vi "Main.vi"() -> ()   [LabVIEW 2017, in "Logger.lvlib"]
doc: "This template is based off of the Queued Message Handler design pattern and the Queued Message Handler project template that ships with LabVIEW.\n\nThe main difference is that the queue is private to this module and communication between modules is performed via Broadcast and Request events.\n\nRequest events are wrapped in public API methods and are handled in the Event Handling Loop (EHL) of this VI. Any module can register for Broadcast events sent by this module. The EHL generates messages based on user interface actions.\n\nThe Message Handling Loop (MHL) processes messages generated by the EHL, or by other messages. The messages are string values, so new messages can be added easily to the Message Cases case structure in the MHL. Each message cluster can also provide an optional value for Message Data, which is a variant that can be converted to whatever message-specific data is required.\n_____\nBased on Delacor QMH Project Template 4.0.0.47.\n_____\nBased on Delacor QMH Project Template 4.1.0.56."
uses:
  Logger.lvlib
  <vilib>/Delacor/Delacor QMH/Libraries/Module Admin_class/Delacor_lib_QMH_Module Admin.lvclass
  Module Data--cluster.ctl
  Stop Argument--cluster.ctl
  <vilib>/Delacor/Delacor QMH/Libraries/Module Admin_class/Delacor_lib_QMH_Module Admin.lvclass/Delacor_lib_QMH_Module Admin.ctl
  Initialize File Argument--cluster.ctl
  Initialize File (Reply Payload)--cluster.ctl
  Log Data Argument--cluster.ctl
  Stop Logging Argument--cluster.ctl
  Settings Editor/Update Application Settings (Reply Payload)--cluster.ctl
  Settings Editor/Settings--cluster.ctl
  CML Shared/Signal Type--enum.ctl
  CML Shared/Calibration Values--cluster.ctl
  <vilib>/Utility/miscctls.llb/LVPointTypeDef.ctl
  <vilib>/Delacor/Delacor QMH/Libraries/Module Admin_class/Delacor_lib_QMH_Get External Launch.vi
  <vilib>/Delacor/Delacor QMH/Libraries/Message Queue_class/Delacor_lib_QMH_Enqueue Message (Single).vi
  <vilib>/Utility/error.llb/Error Cluster From Error Code.vi
  <vilib>/ErrorRing/Error Ring.xnode
  <vilib>/Delacor/Delacor QMH/Libraries/Message Queue_class/Delacor_lib_QMH_Message Queue.lvclass
  Settings Editor/Settings Editor.lvlib
  CML Shared/CML Shared.lvlib
panel:
  out "Settings":T1
  out "error out":errorcluster
  in  "Module Admin":refnum<class "Delacor_lib_QMH_Module Admin.lvclass">
  # "This is a headless module. \nShow its panel to confirm that the Settings are updated correctly and other debugging tasks.\nUse the Settings Editor to change the settings for this module."
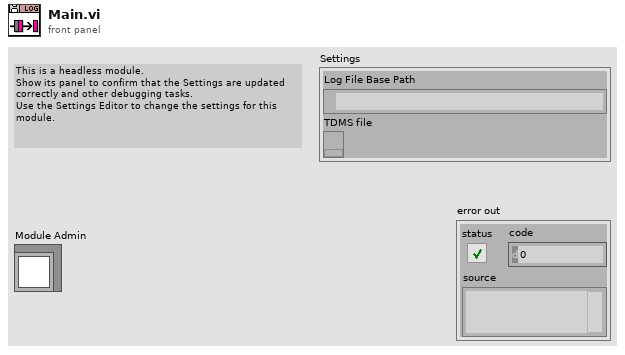
[diagram p1: front panel]
types:
  T1 = typedef "Logger.lvlib/Module Data--cluster.ctl" = cluster{"Log File Base Path":path, "TDMS file":refnum<k34>}
  T2 = typedef "Settings Editor.lvlib/Broadcast Events--cluster.ctl" = cluster{"Module Did Init":refnum<user-event>, "Status Updated":refnum<user-event>, "Error Reported":refnum<user-event>, "Module Did Stop":refnum<user-event>, "Update Module Execution Status":refnum<user-event>, "Application Settings Updated":refnum<user-event>}
  T3 = typedef "Logger.lvlib/Request Events--cluster.ctl" = cluster{"Stop Module":refnum<user-event>, "Show Panel":refnum<user-event>, "Hide Panel":refnum<user-event>, "Get Module Execution Status":refnum<user-event>, "Show Diagram":refnum<user-event>, "Stop Logging":refnum<user-event>, "Log Data":refnum<user-event>, "Initialize File":refnum<user-event>}
  T4 = enum32{"invalid lock state", "Not Locked", "Locked (No Password)", "Password-protected"}
  T5 = typedef "Logger.lvlib/Stop Argument--cluster.ctl" = cluster{"Origin":string, "Exit via Stop Module Req?":bool, "Wait for Module to stop?":bool}
  T6 = typedef "Logger.lvlib/Initialize File Argument--cluster.ctl" = cluster{"Wait Notifier":refnum<notifier>, "wait for reply":bool}
  T7 = typedef "Logger.lvlib/Log Data Argument--cluster.ctl" = cluster{"Waveforms":waveform(dbl)[]}
  T8 = typedef "Logger.lvlib/Stop Logging Argument--cluster.ctl" = cluster{"Boolean":bool}
  T9 = typedef "Settings Editor.lvlib/Update Application Settings (Reply Payload)--cluster.ctl" = cluster{"Settings":T10, "Update Settings_error":errorcluster}
  T10 = typedef "Settings Editor.lvlib/Settings--cluster.ctl" = cluster{"Signal Type":T11, "Calibration Array":T12[], "Log File Base Path":path}
  T11 = typedef "CML Shared.lvlib/Signal Type--enum.ctl" = enum16{"Sine Wave", "Square with Noise"}
  T12 = typedef "CML Shared.lvlib/Calibration Values--cluster.ctl" = cluster{"Slope":dbl, "Offset":dbl}
  T13 = typedef "LVPointTypeDef.ctl" = cluster{"Horizontal":i16, "Vertical":i16}
  T14 = enum32{"Invalid", "Standard", "Closed", "Hidden", "Minimized", "Maximized"}
  T15 = typedef "Logger.lvlib/Initialize File (Reply Payload)--cluster.ctl" = cluster{"File Path":path, "Initialize File_error":errorcluster}
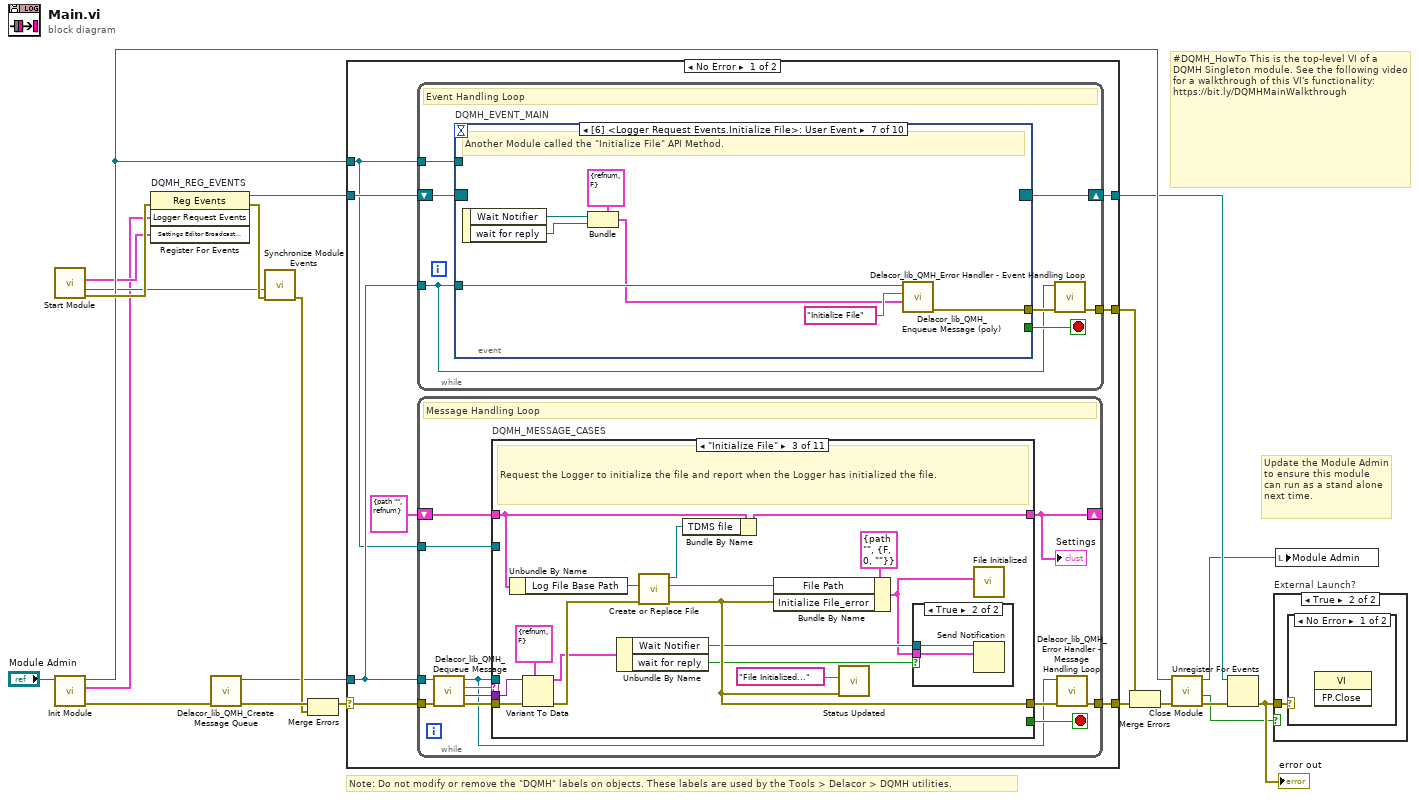
[diagram p0: block diagram]
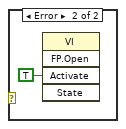
[diagram p3: hidden frame]
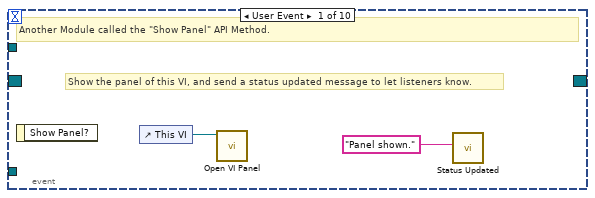
[diagram p4: hidden frame]
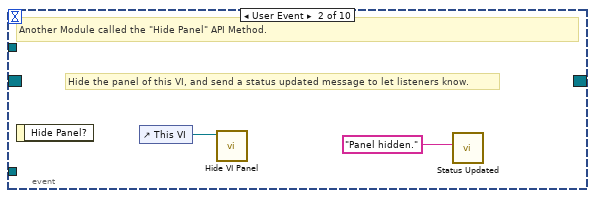
[diagram p5: hidden frame]
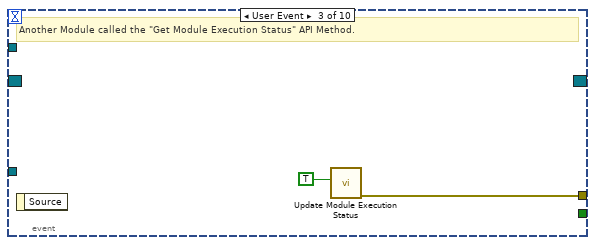
[diagram p6: hidden frame]
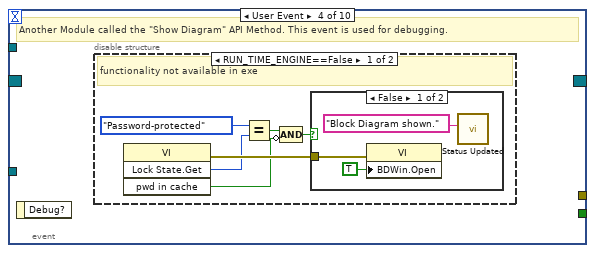
[diagram p7: hidden frame]
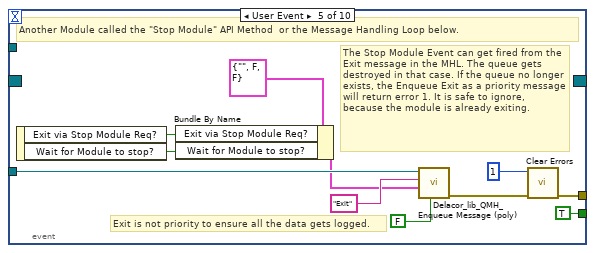
[diagram p10: hidden frame]
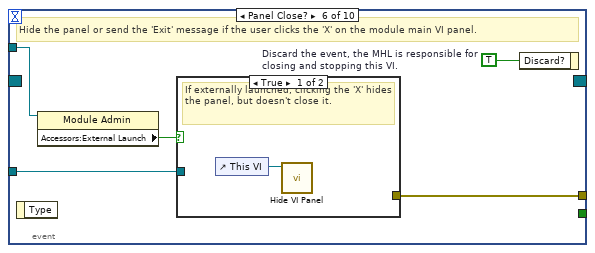
[diagram p11: hidden frame]
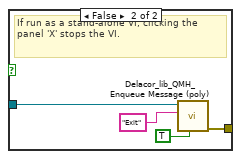
[diagram p12: hidden frame]
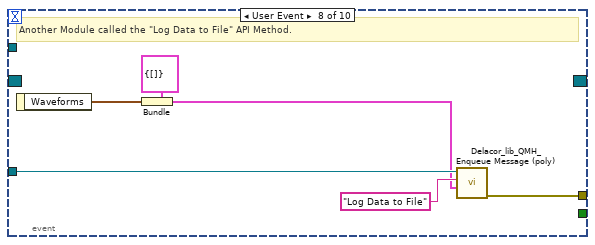
[diagram p13: hidden frame]
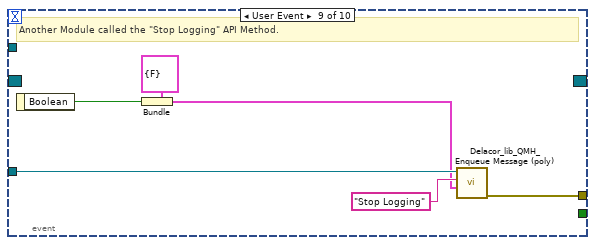
[diagram p14: hidden frame]
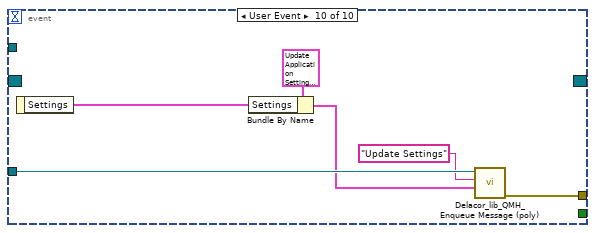
[diagram p15: hidden frame]
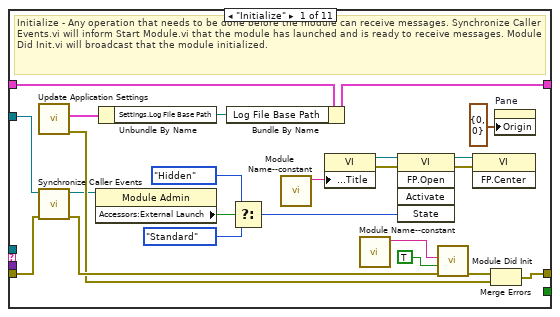
[diagram p16: hidden frame]
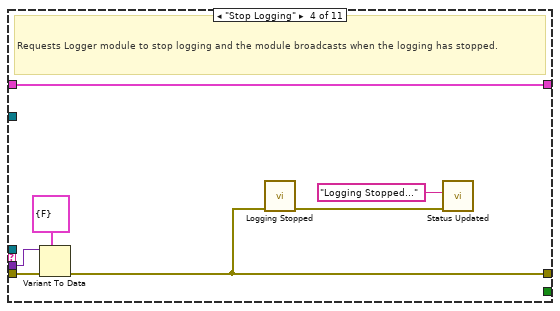
[diagram p19: hidden frame]
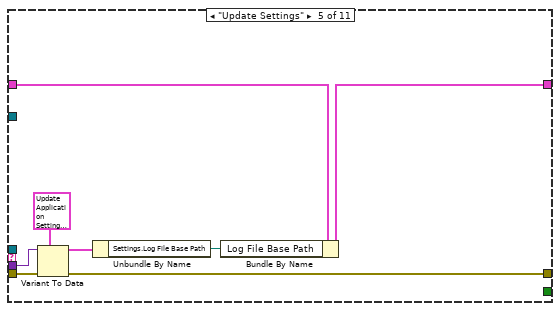
[diagram p20: hidden frame]
diagram:
  # "#DQMH_HowTo This is the top-level VI of a DQMH Singleton module. See the following video for a walkthrough of this VI's functionality: https://bit.ly/DQMHMainWalkthrough"
  # "Note: Do not modify or remove the \"DQMH\" labels on objects. These labels are used by the Tools > Delacor > DQMH utilities."
  # "Update the Module Admin to ensure this module can run as a stand alone next time."
  n1 = call "Start Module.vi"() -> ("error out"=w13:errorcluster, "Wait for Event Sync?"=w3:bool, "Settings Editor Broadcast Events"=w2:T2)  [unwired: 8 in, 1 out]
  n2 = call "Init Module.vi"("Singleton Module Admin in"="Module Admin") -> ("error out"=w20:errorcluster, "Logger Request Events"=w1:T3, "Singleton Module Admin out"=w10:refnum<class "Delacor_lib_QMH_Module Admin.lvclass">)  [unwired: 8 in]
  n3 = register-events "DQMH_REG_EVENTS"(error in=w13, w1, w2) -> (reference out=w8:refnum<event-registration>, error out=w12:errorcluster)  [unwired: 1 in]
  n4 = call <vilib>:"Delacor_lib_QMH_Create Message Queue.vi"("error in (no error)"=w20) -> ("error out"=w15:errorcluster, "Message Queue"=w7:refnum<class "Delacor_lib_QMH_Message Queue.lvclass">)  [unwired: 9 in]
  n5 = call "Synchronize Module Events.vi"("error in (no error)"=w12, "Wait for Event Sync?"=w3) -> ("error out"=w11:errorcluster)  [unwired: 9 in]
  n6 = Merge Errors(w15, w11) -> (w14:errorcluster)
  n7 = case shown="No Error" w14 {
    selector: w14 -> [w27 w235]
    tunnel: [w29 w235] -> w21
    tunnel: [w26 w232] -> w9
    tunnel: w8 -> [w24 w232]
    tunnel: w7 -> [w23 _]
    tunnel: [w28 _] -> w18
    tunnel: w10 -> [w22 w228]
    frame No Error {
      n8 = while {
        tunnel: w23 -> [w30]
        shift-right: [w33] -> w26
        shift-left: w24 -> [w34]
        tunnel: [w35] -> w28
        tunnel: w22 -> [w31]
        stop <- w32 stop-if-true
        # "Event Handling Loop"
        n9 = event "DQMH_EVENT_MAIN" shown="[6] <Logger Request Events.Initialize File>: User Event" {
          selector: w34 -> [_ _ _ _ _ _ _ _ _ _]
          dyn-events: [_ _ _ _ _ _ _ _ _ _] -> w33
          timeout: _ -> [_ _ _ _ _ _ _ _ _ _]
          tunnel: [_ _ _ _ TRUE ("Discard?") _ _ _ _ _] -> w32
          tunnel: w30 -> [_ _ _ _ w58 w65 w78 w84 w90 w96]
          tunnel: [_ _ w42 _ w61 w67 w79 w85 w91 w97] -> w36
          tunnel: w31 -> [_ _ _ _ _ w64 _ _ _ _]
          event User Event {
            # "Show the panel of this VI, and send a status updated message to let listeners know."
            # "Another Module called the \"Show Panel\" API Method."
            n10 = event-data() -> ()  [unwired: 1 in, 1 out]
            n11 = control-ref of="This VI"() -> (w38:refnum<vi>)
            n12 = call "Open VI Panel.vi"("VI"=w38) -> ()  [unwired: 10 in, 1 out]
            n13 = call "Status Updated.vi"("Status"="Panel shown." ("format string")) -> ()  [unwired: 10 in, 1 out]
          }
          event User Event {
            # "Hide the panel of this VI, and send a status updated message to let listeners know."
            # "Another Module called the \"Hide Panel\" API Method."
            n14 = event-data() -> ()  [unwired: 1 in, 1 out]
            n15 = control-ref of="This VI"() -> (w40:refnum<vi>)
            n16 = call "Hide VI Panel.vi"("VI"=w40) -> ()  [unwired: 10 in, 1 out]
            n17 = call "Status Updated.vi"("Status"="Panel hidden." ("format string")) -> ()  [unwired: 10 in, 1 out]
          }
          event User Event {
            # "Another Module called the \"Get Module Execution Status\" API Method."
            n18 = event-data() -> ()  [unwired: 1 in, 1 out]
            n19 = call "Update Module Execution Status.vi"("Running?"=TRUE) -> ("error out"=w42:errorcluster)  [unwired: 10 in]
          }
          event User Event {
            # "Another Module called the \"Show Diagram\" API Method. This event is used for debugging."
            n20 = event-data() -> ()  [unwired: 1 in, 1 out]
            n21 = disable-structure shown="RUN_TIME_ENGINE==False" {
              frame condition #0 (active) {
                # "functionality not available in exe"
                n22 = invoke class="VI" method="Lock State.Get"() -> (error out=w48:errorcluster, "Get Lock State"=w47:T4, "pwd in cache"=w44:bool)  [unwired: 4 in, 1 out]
                n23 = Equal?(x=T4."Password-protected", y=w47) -> (x = y?=w45:bool)
                n24 = Compound Arithmetic op=AND(w45, invert w44) -> (w43:bool)
                n25 = case shown="False" w43 {
                  tunnel: w48 -> [w51 _]
                  frame False {
                    n26 = property class="VI"(error in=w51, "BDWin.Open"=TRUE ("Block Diagram Window:Open")) -> ()  [unwired: 1 in, 2 out]
                    n27 = call "Status Updated.vi"("Status"="Block Diagram shown." ("format string")) -> ()  [unwired: 10 in, 1 out]
                  }
                  frame True {
                    # "Password-protected VI, and the password is not in the cache. Do not show the diagram."
                  }
                }
              }
              frame condition #1 {
              }
            }
          }
          event User Event {
            # "Exit is not priority to ensure all the data gets logged."
            # "The Stop Module Event can get fired from the Exit message in the MHL. The queue gets destroyed in that case. If the queue no longer exists, the Enqueue Exit as a priority message will return error 1. It is safe to ignore, because the module is already exiting."
            # "Another Module called the \"Stop Module\" API Method  or the Message Handling Loop below."
            n28 = event-data() -> ("Exit via Stop Module Req?"=w54:bool, "Wait for Module to stop?"=w53:bool)  [unwired: 1 in]
            n29 = Bundle By Name(cluster=T5 {"Origin"="", "Exit via Stop Module Req?"=FALSE, "Wait for Module to stop?"=FALSE} ("Stop Argument"), "Exit via Stop Module Req?"=w54, "Wait for Module to stop?"=w53) -> (w52:T5)
            n30 = call-poly <vilib>:"Delacor_lib_QMH_Enqueue Message (poly).vi"("Priority Message? (F)"=FALSE, "Message Data"=w52, "Message"="Exit", "Message Queue in"=w58) -> ("error out"=w62:errorcluster)  [unwired: 6 in, 1 out]
            n31 = call <vilib>:"Clear Errors.vi"("error in (no error)"=w62, "specific error code to clear (0: all)"=1) -> ("error out"=w61:errorcluster)  [unwired: 4 in, 1 out]
          }
          event Panel Close? {
            w66 = TRUE  # Discard the event, the MHL is responsible for closing and stopping this VI.
            # "Hide the panel or send the 'Exit' message if the user clicks the 'X' on the module main VI panel."
            n32 = event-data() -> ()  [unwired: 1 in, 1 out]
            n33 = property class="Module Admin"(reference=w64) -> ("Accessors:External Launch"=w63:bool)  [unwired: 1 in, 2 out]
            n34 = case shown="True" w63 {
              tunnel: w65 -> [_ w71]
              tunnel: [_ w72] -> w67
              frame True {
                # "If externally launched, clicking the 'X' hides the panel, but doesn't close it."
                n35 = control-ref of="This VI"() -> (w68:refnum<vi>)
                n36 = call "Hide VI Panel.vi"("VI"=w68) -> ()  [unwired: 10 in, 1 out]
              }
              frame False {
                # "If run as a stand-alone VI, clicking the panel 'X' stops the VI."
                n37 = call-poly <vilib>:"Delacor_lib_QMH_Enqueue Message (poly).vi"("Priority Message? (F)"=TRUE, "Message"="Exit", "Message Queue in"=w71) -> ("error out"=w72:errorcluster)  [unwired: 7 in, 1 out]
              }
            }
            n38 = event-data("Discard?"=w66) -> ()  [unwired: 1 in, 1 out]
          }
          event User Event {
            # "Another Module called the \"Initialize File\" API Method."
            n39 = event-data() -> ("Wait Notifier"=w74:refnum<notifier>, "wait for reply"=w73:bool)  [unwired: 1 in]
            n40 = Bundle(cluster=T6 {"Wait Notifier"=refnum, "wait for reply"=FALSE} ("Initialize File Argument"), "Wait Notifier"=w74, "wait for reply"=w73) -> (w75:T6)
            n41 = call-poly <vilib>:"Delacor_lib_QMH_Enqueue Message (poly).vi"("Message Data"=w75, "Message"="Initialize File", "Message Queue in"=w78) -> ("error out"=w79:errorcluster)  [unwired: 7 in, 1 out]
          }
          event User Event {
            # "Another Module called the \"Log Data to File\" API Method."
            n42 = event-data() -> ("Waveforms"=w80:waveform(dbl)[])  [unwired: 1 in]
            n43 = Bundle(cluster=T7 {"Waveforms"=[]} ("Log Data to File Argument"), "Waveforms"=w80) -> (w81:T7)
            n44 = call-poly <vilib>:"Delacor_lib_QMH_Enqueue Message (poly).vi"("Message Data"=w81, "Message"="Log Data to File", "Message Queue in"=w84) -> ("error out"=w85:errorcluster)  [unwired: 7 in, 1 out]
          }
          event User Event {
            # "Another Module called the \"Stop Logging\" API Method."
            n45 = event-data() -> ("Boolean"=w86:bool)  [unwired: 1 in]
            n46 = Bundle(cluster=T8 {"Boolean"=FALSE} ("Stop Logging Argument"), "Boolean"=w86) -> (w87:T8)
            n47 = call-poly <vilib>:"Delacor_lib_QMH_Enqueue Message (poly).vi"("Message Data"=w87, "Message"="Stop Logging", "Message Queue in"=w90) -> ("error out"=w91:errorcluster)  [unwired: 7 in, 1 out]
          }
          event User Event {
            n48 = event-data() -> ("Settings"=w93:T10)  [unwired: 1 in]
            n49 = Bundle By Name(cluster=T9 {"Settings"={"Signal Type"=enum."Sine Wave", "Calibration Array"=[], "Log File Base Path"=path ""}, "Update Settings_error"={"status"=FALSE, "code"=0, "source"=""}} ("Settings Updated Argument"), "Settings"=w93) -> (w92:T9)
            n50 = call-poly <vilib>:"Delacor_lib_QMH_Enqueue Message (poly).vi"("Message Data"=w92, "Message"="Update Settings", "Message Queue in"=w96) -> ("error out"=w97:errorcluster)  [unwired: 7 in, 1 out]
          }
        }
        n51 = call-dynamic "Delacor_lib_QMH_Error Handler - Event Handling Loop.vi"("error in (no error)"=w36, "Message Queue in"=w30) -> ("dup error in"=w35:errorcluster)  [unwired: 8 in, 1 out]
      }
      n52 = while {
        tunnel: w23 -> [w100]
        shift-right: [w104] -> _
        shift-left: T1 {"Log File Base Path"=path "", "TDMS file"=refnum} ("Data Cluster") -> [w105]
        tunnel: w27 -> [w108]
        tunnel: [w106] -> w29
        tunnel: w22 -> [w98]
        stop <- w103 stop-if-true
        # "Message Handling Loop"
        n53 = call-dynamic "Delacor_lib_QMH_Dequeue Message.vi"("error in (no error)"=w108, "Message Queue in"=w100) -> ("error out"=w107:errorcluster, "Message Data"=w101:variant, "Message"=w102:string, "Message Queue out"=w99:refnum<class "Delacor_lib_QMH_Message Queue.lvclass">)  [unwired: 6 in]
        n54 = case "DQMH_MESSAGE_CASES" shown="\"Initialize File\"" w102 {
          selector: w102 -> [_ _ _ _ _ _ _ _ _ _ w215]
          tunnel: w99 -> [_ _ _ _ _ _ _ _ w184 w207 _]
          tunnel: w107 -> [w130 w134 w150 w159 w167 w176 w179 w181 w191 w213 w217]
          tunnel: [w127 w134 w149 w158 w166 w174 w178 w181 w187 w210 w218] -> w109
          tunnel: w105 -> [w117 w133 w138 w154 w165 w169 w177 w180 w186 w199 w216]
          tunnel: [w111 w133 w137 w154 w163 w169 w177 w180 w186 w199 w216] -> w104
          tunnel: [_ _ _ _ _ _ _ _ _ w206 _] -> w103
          tunnel: w101 -> [_ _ w147 w156 w164 w173 _ _ w185 w205 _]
          tunnel: w98 -> [w118 _ _ _ _ _ _ _ w183 w200 _]
          frame "Initialize" {
            # "Initialize - Any operation that needs to be done before the module can receive messages. Synchronize Caller Events.vi will inform Start Module.vi that the module has launched and is ready to receive messages. Module Did Init.vi will broadcast that the module initialized."
            n55 = call "Update Application Settings.vi"() -> ("error out"=w126:errorcluster, "Reply Payload"=w112:T9)  [unwired: 9 in, 1 out]
            n56 = call "Synchronize Caller Events.vi"("error in (no error)"=w130, "Singleton Module Admin in"=w118) -> ("error out"=w129:errorcluster, "Singleton Module Admin out"=w114:refnum<class "Delacor_lib_QMH_Module Admin.lvclass">)  [unwired: 8 in]
            n57 = property class="Module Admin"(reference=w114) -> ("Accessors:External Launch"=w122:bool)  [unwired: 1 in, 2 out]
            n58 = Unbundle By Name(w112) -> ("Settings.Log File Base Path"=w110:path)
            n59 = Bundle By Name(cluster=w117, "Log File Base Path"=w110) -> (w111:T1)
            n60 = Select(t=T14."Hidden" ("State"), s=w122, f=T14."Standard" ("State")) -> (s? t:f=w119:T14)
            n61 = call "Module Name--constant.vi"() -> ("Module Name"=w125:string)  [unwired: 11 in]
            n62 = property class="VI"("Front Panel.Title"=w125) -> (reference out=w124:refnum<vi>, error out=w132:errorcluster)  [unwired: 2 in]
            n63 = call "Module Name--constant.vi"() -> ("Module Name"=w115:string)  [unwired: 11 in]
            n64 = invoke class="VI" method="FP.Open"(reference=w124, error in=w132, "State"=w119) -> (reference out=w123:refnum<vi>, error out=w131:errorcluster)  [unwired: 2 in, 3 out]
            n65 = call "Module Did Init.vi"("error in (no error)"=w129, "Initialized?"=TRUE, "Origin"=w115) -> ("error out"=w128:errorcluster)  [unwired: 8 in]
            n66 = invoke class="VI" method="FP.Center"(reference=w123, error in=w131) -> ()  [unwired: 1 in, 3 out]
            n67 = Merge Errors(w128, w126) -> (w127:errorcluster)
            n68 = property on="Pane" class="Pane"("Origin"=T13 {"Horizontal"=0, "Vertical"=0}) -> ()  [unwired: 2 in, 2 out]
          }
          frame "--- Module Specific ---" {
            # "Separator -- The following cases handle messages specific to this Module."
          }
          frame "Initialize File" {
            # "Request the Logger to initialize the file and report when the Logger has initialized the file."
            n69 = Unbundle By Name(w138) -> ("Log File Base Path"=w140:path)
            n70 = Variant To Data(error in=w150, type=T6 {"Wait Notifier"=refnum, "wait for reply"=FALSE} ("Initialize File Argument"), Variant=w147) -> (data=w145:T6, error out=w148:errorcluster)
            n71 = Unbundle By Name(w145) -> ("Wait Notifier"=w144:refnum<notifier>, "wait for reply"=w143:bool)
            n72 = call "Create or Replace File.vi"("error in (no error)"=w148, "Log File Base Path"=w140) -> ("error out"=w149:errorcluster, "File Path"=w136:path, "Refnum out"=w139:refnum<k34>)  [unwired: 7 in]
            n73 = Bundle By Name(cluster=w138, "TDMS file"=w139) -> (w137:T1)
            n74 = Bundle By Name(cluster=T15 {"File Path"=path "", "Initialize File_error"={"status"=FALSE, "code"=0, "source"=""}} ("Initialize File (Reply Payload)"), "File Path"=w136, "Initialize File_error"=w149) -> (w141:T15)
            n75 = call "Status Updated.vi"("error in (no error)"=w149, "Status"="File Initialized...") -> ()  [unwired: 9 in, 1 out]
            n76 = case shown="True" w143 {
              tunnel: w144 -> [_ w152]
              tunnel: w141 -> [_ w151]
              frame False {
              }
              frame True {
                n77 = Send Notification(notification=w151, notifier=w152) -> ()  [unwired: 1 in, 2 out]
              }
            }
            n78 = call "File Initialized.vi"("Reply Payload"=w141) -> ()  [unwired: 10 in, 1 out]
          }
          frame "Stop Logging" {
            # "Requests Logger module to stop logging and the module broadcasts when the logging has stopped."
            n79 = Variant To Data(error in=w159, type=T8 {"Boolean"=FALSE} ("Stop Logging Argument"), Variant=w156) -> (error out=w158:errorcluster)  [unwired: 1 out]
            n80 = call "Logging Stopped.vi"("error in (no error)"=w158) -> ("error out"=w157:errorcluster)  [unwired: 10 in]
            n81 = call "Status Updated.vi"("error in (no error)"=w157, "Status"="Logging Stopped...") -> ()  [unwired: 9 in, 1 out]
          }
          frame "Update Settings" {
            n82 = Variant To Data(error in=w167, type=T9 {"Settings"={"Signal Type"=enum."Sine Wave", "Calibration Array"=[], "Log File Base Path"=path ""}, "Update Settings_error"={"status"=FALSE, "code"=0, "source"=""}} ("Settings Updated Argument"), Variant=w164) -> (data=w162:T9, error out=w166:errorcluster)
            n83 = Unbundle By Name(w162) -> ("Settings.Log File Base Path"=w161:path)
            n84 = Bundle By Name(cluster=w165, "Log File Base Path"=w161) -> (w163:T1)
          }
          frame "Log Data to File" {
            # "Requests Logger module to log data to file"
            n85 = Variant To Data(error in=w176, type=T7 {"Waveforms"=[]} ("Log Data to File Argument"), Variant=w173) -> (data=w171:T7, error out=w175:errorcluster)
            n86 = Unbundle By Name(w169) -> ("TDMS file"=w168:refnum<k34>)
            n87 = Unbundle By Name(w171) -> ("Waveforms"=w170:waveform(dbl)[])
            n88 = call "Log Data to File.vi"("error in (no error)"=w175, "Data to log"=w170, "TDMS File Reference"=w168) -> ("error out"=w174:errorcluster)  [unwired: 8 in]
          }
          frame "---Copy This Frame---" {
            # "Duplicate this frame when creating new messages.  Change this comment in the duplicated frame to describe this message."
            n89 = Merge Errors(w179) -> (w178:errorcluster)
          }
          frame "--- Exit and Error Handling---" {
            # "Separator - The following cases handle errors and exit messages."
          }
          frame "Error" {
            # "Error - Check the error message data and respond accordingly. This message is sent by the \"Error Handler\" VIs at the end of each loop in this application."
            n90 = property class="Module Admin"(reference=w183) -> ("Accessors:External Launch"=w182:bool)  [unwired: 1 in, 2 out]
            n91 = Variant To Data(error in=w191, type=errorcluster {"status"=FALSE, "code"=0, "source"=""} ("error constant"), Variant=w185) -> (data=w192:errorcluster, error out=w189:errorcluster)
            n92 = call "Error Reported.vi"("Error"=w192) -> ()  [unwired: 10 in, 1 out]
            n93 = case shown="False" w182 {
              tunnel: [w197 _] -> w188
              tunnel: w184 -> [w195 _]
              tunnel: w192 -> [w196 _]
              frame False {
                # "If the module is running standalone, then pop up an error dialog and call the \"Exit\" message."
                n94 = call <vilib>:"Simple Error Handler.vi"("error in (no error)"=w196) -> ()  [unwired: 4 in, 5 out]
                n95 = call-poly <vilib>:"Delacor_lib_QMH_Enqueue Message (poly).vi"("Priority Message? (F)"=TRUE, "Message"="Exit", "Message Queue in"=w195) -> ("error out"=w197:errorcluster)  [unwired: 7 in, 1 out]
              }
              frame True {
                # "If the module was launched externally, calling the Error Reported broadcast VI is the only action performed by the \"Error\" message. The module's caller can then process the error appropriately."
              }
            }
            n96 = Merge Errors(w189, w188) -> (w187:errorcluster)
            n97 = local write "error out"(w187) -> ()
          }
          frame "Exit" {
            w204 = 91  # 91: not all Exit messages will have an argument
            w206 = TRUE  # Stop the VI
            # "Release the message queue reference"
            # "Exit - Exit the application."
            n98 = Variant To Data(error in=w213, type=T5 {"Origin"="", "Exit via Stop Module Req?"=FALSE, "Wait for Module to stop?"=FALSE} ("Stop Argument"), Variant=w205) -> (data=w202:T5, error out=w209:errorcluster)
            n99 = Unbundle By Name(w199) -> ("TDMS file"=w198:refnum<k34>)
            n100 = call <vilib>:"Clear Errors.vi"("error in (no error)"=w209, "specific error code to clear (0: all)"=w204) -> ("error out"=w212:errorcluster)  [unwired: 4 in, 1 out]
            n101 = control-ref of="This VI"() -> (w201:refnum<vi>)
            n102 = call-dynamic "Delacor_lib_QMH_Release Message Queue.vi"("error in (no error)"=w212, "Message Queue"=w207) -> ("error out"=w211:errorcluster)  [unwired: 9 in]
            n103 = call "Handle Exit.vi"("Stop Argument"=w202, "Admin in"=w200, "VI reference"=w201) -> ("error out"=w208:errorcluster)  [unwired: 7 in, 1 out]
            n104 = call "Close File.vi"("Refnum out"=w198) -> ()  [unwired: 10 in, 1 out]
            n105 = Merge Errors(w211, w208) -> (w210:errorcluster)
          }
          frame Default {
            # "'Default' case only runs if there is a message that isn't defined in any of the other cases.  Output a programming error."
            n106 = call "Module Name--constant.vi"() -> ("Module Name"=w214:string)  [unwired: 11 in]
            n107 = xnode "Error Ring"("parameter 0"=w215, "parameter 1"=w214) -> ("error out"=w219:errorcluster)
            n108 = Merge Errors(w217, w219) -> (w218:errorcluster)
          }
        }
        "Settings" <- w104
        n109 = call-dynamic "Delacor_lib_QMH_Error Handler - Message Handling Loop.vi"("error in (no error)"=w109, "Message Queue in"=w99) -> ("dup error in"=w106:errorcluster)  [unwired: 8 in, 1 out]
      }
    }
    frame Error {
      # "Synchronize Caller Events.vi will inform Start Module.vi that the module has launched and will let the code calling Start Module.vi register for broadcasts and would permit the caller receive the broadcast that an error occurred at launch time."
      n110 = call "Synchronize Caller Events.vi"("Singleton Module Admin in"=w228) -> ("error out"=w233:errorcluster)  [unwired: 9 in, 1 out]
      n111 = call "Module Name--constant.vi"() -> ("Module Name"=w231:string)  [unwired: 11 in]
      n112 = Format Into String(format string="An error occurred during initialization. %s is no longer running.", w231) -> (resulting string=w229:string)  [unwired: 2 in, 1 out]
      n113 = Merge Errors(w235, w233) -> (w234:errorcluster)
      n114 = call "Error Reported.vi"("Additional Information"=w229, "Error"=w234) -> ()  [unwired: 9 in, 1 out]
    }
  }
  n115 = Merge Errors(w18, w21) -> (w17:errorcluster)
  n116 = call "Close Module.vi"("error in (no error)"=w17, "Module Admin in"=w10) -> ("error out"=w19:errorcluster, "External Launch"=w4:bool, "Module Admin out"=w5:refnum<class "Delacor_lib_QMH_Module Admin.lvclass">)  [unwired: 7 in]
  n117 = Unregister For Events(event registration refnum=w9, error in=w19) -> (error out=w16:errorcluster)
  "error out" <- w16
  n118 = case "External Launch?" shown="True" w4 {
    tunnel: w16 -> [_ w236]
    frame False {
    }
    frame True {
      n119 = case shown="No Error" w236 {
        frame No Error {
          n120 = invoke class="VI" method="FP.Close"() -> ()  [unwired: 3 in, 3 out]
        }
        frame Error {
          n121 = invoke class="VI" method="FP.Open"("Activate"=TRUE ("Activate?")) -> ()  [unwired: 4 in, 5 out]
        }
      }
    }
  }
  n122 = local write "Module Admin"(w5) -> ()
